vi "Read Insert.vi"(8 "error in (no error)":errorcluster, 11 "Insert_STR in":refnum<class "Insert_STR.lvclass">=refnum) -> (0 "error out":errorcluster, 2 "Abs_Value.lvclass":refnum<class "Abs_Value.lvclass">, 3 "Insert_STR out":refnum<class "Insert_STR.lvclass">)   [LabVIEW 2021, in "Insert_STR.lvclass"]
uses:
  Insert_STR.lvclass
  Abs_Types/Value/Abs_Value.lvclass
  C:/New folder/LV_Abstract/LV_Abstract/Source/Abs_Types/Type/Abs_Type.lvclass
  C:/New folder/LV_Abstract/LV_Abstract/Source/Abs_Types/Value/Abs_Value.lvclass
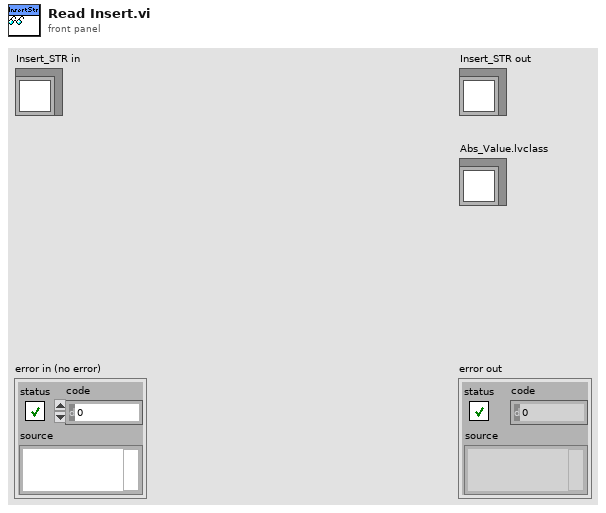
[diagram p1: front panel]
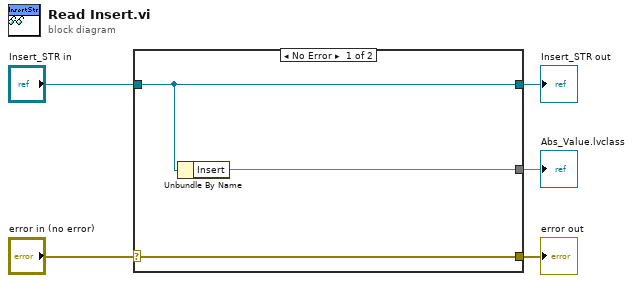
[diagram p0: block diagram]
diagram:
  n1 = case shown="No Error" "error in (no error)" {
    selector: "error in (no error)" -> [w8 w9]
    tunnel: [w8 w9] -> w4
    tunnel: [w7 w10] -> w2
    tunnel: "Insert_STR in" -> [w7 w10]
    tunnel: [w6 _] -> w1
    frame No Error {
      n2 = Unbundle By Name(w7) -> ("Insert"=w6)
    }
    frame Error {
    }
  }
  "error out" <- w4
  "Insert_STR out" <- w2
  "Abs_Value.lvclass" <- w1
